vi "禹山浊度_获取用户校准参数.vi"(8 "error in (no error)":errorcluster caption="错误输入（无错误）", 11 "MB session in":refnum<class "MB_Master.lvclass">) -> (0 "error out":errorcluster caption="错误输出", 2 "输出值":cluster{"K":sgl, "B":sgl}, 3 "MB session out":refnum<class "MB_Master.lvclass">)   [LabVIEW 2016, in "斯坦道多参数.lvlib"]
uses:
  <vilib>/Plasmionique/MB Master/MB_Master/MB_Master.lvclass
  <vilib>/Plasmionique/MB Master/MB Master.lvlib
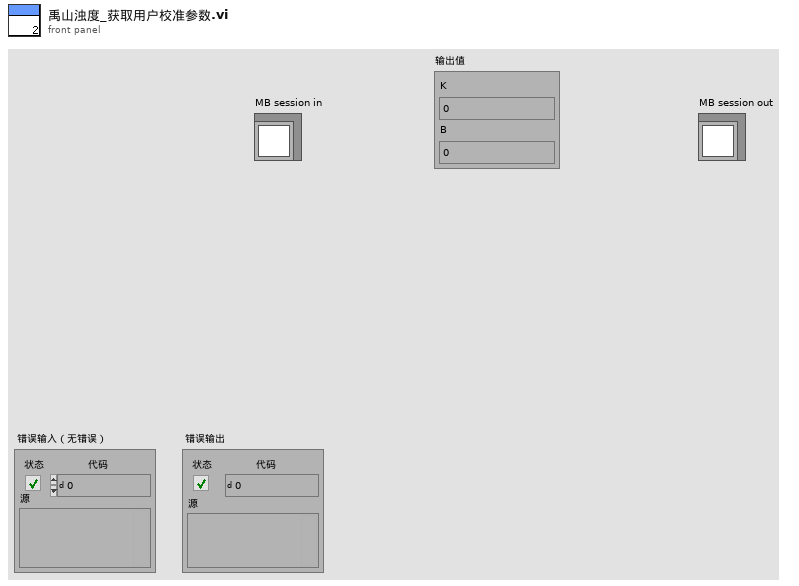
[diagram p1: front panel]
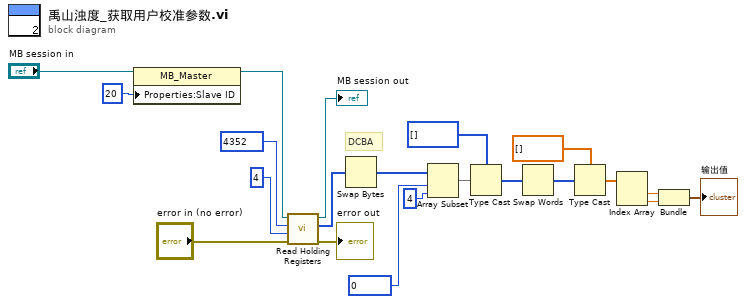
[diagram p0: block diagram]
diagram:
  # "DCBA"
  n1 = property class="MB_Master"(reference="MB session in", "Properties:Slave ID"=u16 20 ("y")) -> (reference out=w9:refnum<class "MB_Master.lvclass">)  [unwired: 1 in, 1 out]
  n2 = call <vilib>:"Read Holding Registers.vi"("error in (no error)"="error in (no error)", "quantity"=u16 4, "starting address"=u16 4352, "MB session in"=w9) -> ("error out"=→"error out":errorcluster, "Registers"=w6:u16[], "MB session out"=→"MB session out":refnum<class "MB_Master.lvclass">)  [unwired: 5 in]
  n3 = Swap Bytes(anything=w6) -> (byte swapped=w5:u16[])
  n4 = Array Subset(array=w5, index=u16 0 ("starting address"), length=4 ("长度")) -> (w4:u16[])
  n5 = Type Cast(type=u32[] [] ("数组 2"), x=w4) -> (*(type *) &x=w16:u32[])
  n6 = Swap Words(1:w16) -> (0:w18:u32[])
  n7 = Type Cast(type=sgl[] [] ("数组 2"), x=w18) -> (*(type *) &x=w14:sgl[])
  n8 = Index Array(array=w14) -> (element #1=w13:sgl, element #2=w12:sgl)  [unwired: 2 in]
  n9 = Bundle("数值"=w13, "数值"=w12) -> (→"输出值":cluster{"数值":sgl, "数值":sgl})  [unwired: 1 in]
